vi "FRCts20_Backend_Test_Request_Delete.vi"(8 "error in (no error)":errorcluster, 11 "Request Index":u32) -> (0 "error out":errorcluster, 1 "Time (ms)":u32, 2 "Status":string, 3 "Request Out":T1, 5 "Success":bool)   [LabVIEW 2014, in "FRCts20_Backend_TestCode.lvlib"]
uses:
  FRCts20_Backend_TestCode.lvlib
  FRCts20_Backend_API/FRCts20_Backend_API_Request.ctl
  FRCts20_Backend_API/FRCts20_Backend_API_Status.ctl
  FRCts20_Backend_API/FRCts20_Backend_API_Command_Request.ctl
  FRCts20_Backend_API/FRCts20_Backend_API_Request.vi
  FRCts20_Backend_API/FRCts20_Backend_API.lvlib
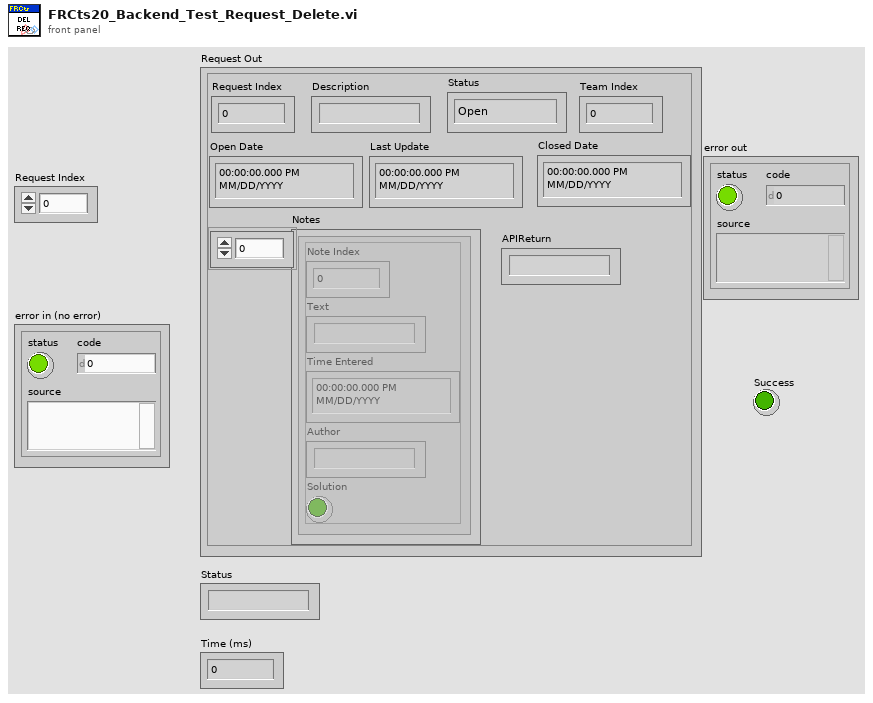
[diagram p1: front panel]
types:
  T1 = typedef "FRCts20_Backend_API.lvlib/FRCts20_Backend_API_Request.ctl" = cluster{"Request Index":u32, "Description":string, "Status":T2, "Open Date":timestamp, "Last Update":timestamp, "Closed Date":timestamp, "Notes":cluster{"Note Index":u32, "Text":string, "Time Entered":timestamp, "Author":string, "Solution":bool}[], "Team Index":u32, "APIReturn":string}
  T2 = typedef "FRCts20_Backend_API.lvlib/FRCts20_Backend_API_Status.ctl" = enum16{"Open", "In Work", "Closed"}
  T3 = typedef "FRCts20_Backend_API.lvlib/FRCts20_Backend_API_Command_Request.ctl" = string
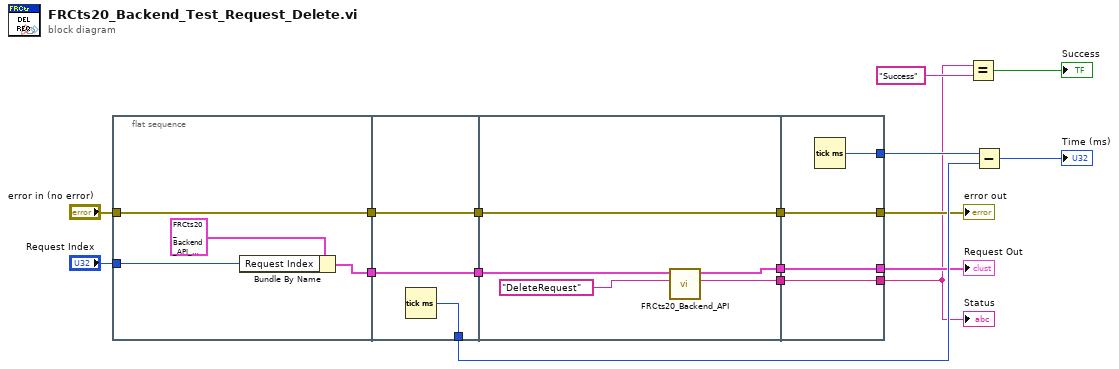
[diagram p0: block diagram]
diagram:
  n1 = flat-sequence {
    tunnel: [w21] -> w17
    tunnel: [w19] -> w16
    tunnel: "error in (no error)" -> [w19]
    tunnel: "Request Index" -> [w18]
    tunnel: w17 -> [w24]
    tunnel: [w24] -> w15
    tunnel: [w23] -> w7
    tunnel: [w22] -> w14
    tunnel: w16 -> [w22]
    tunnel: w15 -> [w28]
    tunnel: [w27] -> w13
    tunnel: [w26] -> w12
    tunnel: w14 -> [w25]
    tunnel: [w25] -> w11
    tunnel: w13 -> [w33]
    tunnel: w12 -> [w32]
    tunnel: [w33] -> w1
    tunnel: [w32] -> w5
    tunnel: [w31] -> w8
    tunnel: [w30] -> w4
    tunnel: w11 -> [w30]
    frame #0 {
      n2 = Bundle By Name(cluster=T1 {"Request Index"=0, "Description"="", "Status"=enum."Open", "Open Date"=timestamp(0 s since 1904-01-01), "Last Update"=timestamp(0 s since 1904-01-01), "Closed Date"=timestamp(0 s since 1904-01-01), "Notes"=[], "Team Index"=0, "APIReturn"=""} ("Request In"), "Request Index"=w18) -> (w21:T1)
    }
    frame #1 {
      n3 = Tick Count (ms)() -> (millisecond timer value=w23:u32)
    }
    frame #2 {
      n4 = call-poly "FRCts20_Backend_API.vi"("Command"=T3 "DeleteRequest", "Request In"=w28) -> ("Status"=w27:string, "Request Out"=w26:T1)  [unwired: 7 in, 1 out]
    }
    frame #3 {
      n5 = Tick Count (ms)() -> (millisecond timer value=w31:u32)
    }
  }
  n6 = Equal?(x=w1, y="Success") -> (x = y?=→"Success":bool)
  n7 = Subtract(x=w8, y=w7) -> (x-y=→"Time (ms)":u32)
  "Status" <- w1
  "Request Out" <- w5
  "error out" <- w4
